vi "Rate scan x8.vi"(6 "T Ventana":u32 format="%x", 7 "Espera acceso USB":u32, 8 "error in 2":errorcluster, 9 "Valor buscado scalers (5000)":u16, 10 "Sumador":u8, 11 "ftHandle_in 2":u32) -> (0 "error out 2":errorcluster, 1 "DAC\nTH3,TH4,TH5":u16, 2 "DAC\nTH0,TH1,TH2":u16, 3 "ftHandle_out 2":u32, 5 "Scaler 1":u16)   [LabVIEW 2009]
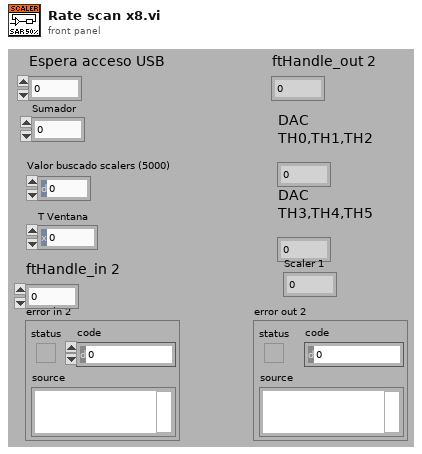
[diagram p1: front panel]
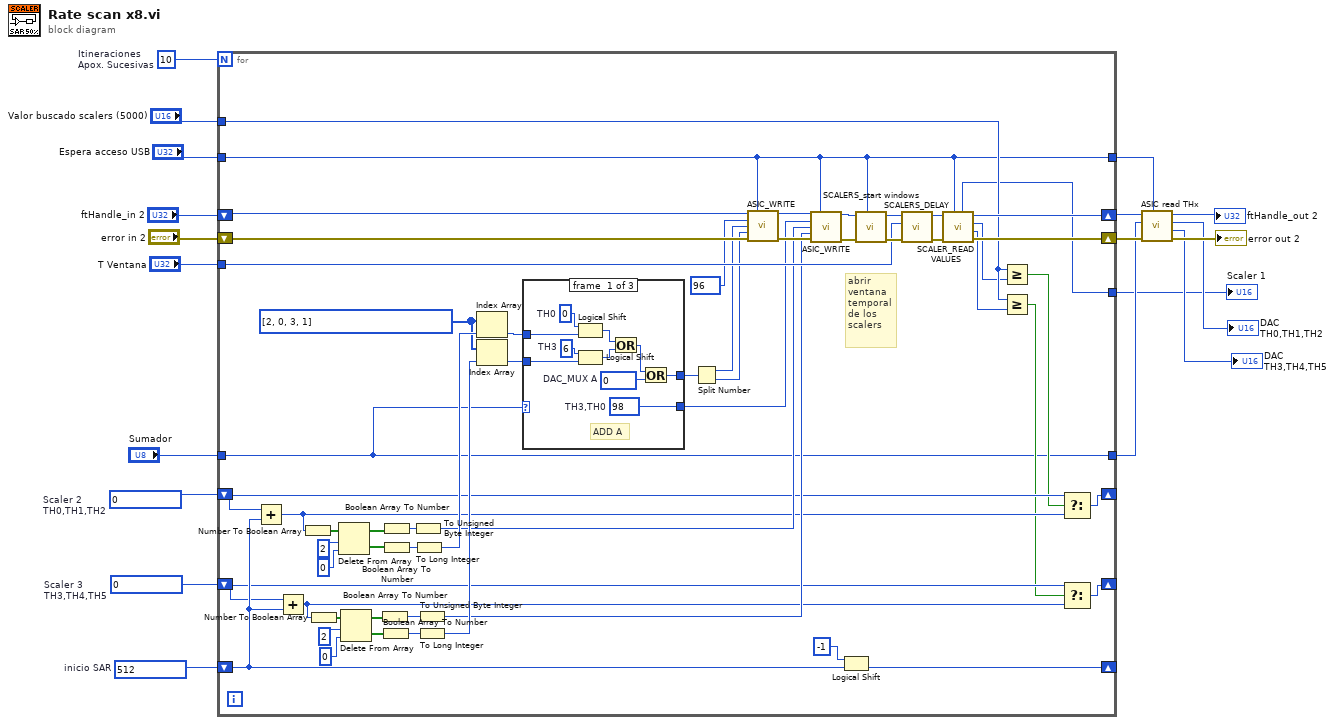
[diagram p0: block diagram]
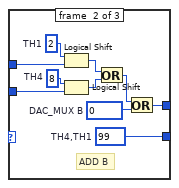
[diagram p2: hidden frame]
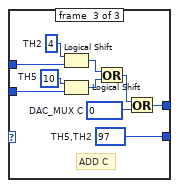
[diagram p3: hidden frame]
diagram:
  w11 = u16 0  # Scaler 3 TH3,TH4,TH5
  w12 = u16 0  # Scaler 2 TH0,TH1,TH2
  w13 = u16 512  # inicio SAR
  w15 = 10  # Itineraciones Apox. Sucesivas
  n1 = for {
    N: w15 -> [_]
    tunnel: "Espera acceso USB" -> [w21]
    tunnel: "T Ventana" -> [w73]
    tunnel: "Valor buscado scalers (5000)" -> [w23]
    shift-right: [w69] -> _
    shift-left: w13 -> [w68]
    shift-right: [w28] -> _
    shift-left: w12 -> [w35]
    shift-right: [w27] -> _
    shift-left: w11 -> [w33]
    tunnel: "Sumador" -> [w25]
    shift-right: [w30] -> w8
    shift-left: "ftHandle_in 2" -> [w51]
    shift-right: [w29] -> w9
    shift-left: "error in 2" -> [w50]
    tunnel: [w25] -> w6
    tunnel: [w21] -> w7
    tunnel: [w20] -> w1
    w48 = u16[] [2, 0, 3, 1]
    # "abrir ventana temporal de los scalers"
    n2 = Add(x=w35, y=w68) -> (x+y=w34:u16)
    n3 = Add(x=w33, y=w68) -> (x+y=w32:u16)
    n4 = Number To Boolean Array(number=w34) -> (Boolean array=w67:bool[])
    n5 = Number To Boolean Array(number=w32) -> (Boolean array=w66:bool[])
    n6 = Delete From Array(array=w67, length=2, index=0) -> (deleted portion=w60:bool[], array with subset deleted=w65:bool[])
    n7 = Delete From Array(array=w66, length=2, index=0) -> (deleted portion=w58:bool[], array with subset deleted=w59:bool[])
    n8 = Boolean Array To Number(Boolean array=w59) -> (number=w56:u32)
    n9 = Boolean Array To Number(Boolean array=w58) -> (number=w54:u32)
    n10 = Boolean Array To Number(Boolean array=w65) -> (number=w57:u32)
    n11 = Boolean Array To Number(Boolean array=w60) -> (number=w55:u32)
    n12 = To Unsigned Byte Integer(number=w57) -> (unsigned 8bit integer=w39:u8)
    n13 = To Long Integer(number=w55) -> (32bit integer=w53:i32)
    n14 = To Unsigned Byte Integer(number=w56) -> (unsigned 8bit integer=w38:u8)
    n15 = To Long Integer(number=w54) -> (32bit integer=w52:i32)
    n16 = Index Array(array=w48, index=w53) -> (element=w47:u16)
    n17 = Index Array(array=w48, index=w52) -> (element=w46:u16)
    n18 = case shown="0, Default" w25 {
      tunnel: [w85 w95 w105] -> w40
      tunnel: w47 -> [w84 w94 w104]
      tunnel: w46 -> [w83 w93 w103]
      tunnel: [w77 w87 w97] -> w41
      frame #0 {
        w76 = u16 0  # DAC_MUX A
        w81 = i8 6  # TH3
        w82 = i8 0  # TH0
        w85 = u8 98  # TH3,TH0
        # "ADD A"
        n19 = Logical Shift(y=w82, x=w84) -> (x << y=w79:u16)
        n20 = Logical Shift(y=w81, x=w83) -> (x << y=w80:u16)
        n21 = Or(x=w79, y=w80) -> (x .or. y?=w78:u16)
        n22 = Or(x=w78, y=w76) -> (x .or. y?=w77:u16)
      }
      frame #1 {
        w86 = u16 0  # DAC_MUX B
        w91 = i8 8  # TH4
        w92 = i8 2  # TH1
        w95 = u8 99  # TH4,TH1
        # "ADD B"
        n23 = Logical Shift(y=w92, x=w94) -> (x << y=w89:u16)
        n24 = Logical Shift(y=w91, x=w93) -> (x << y=w90:u16)
        n25 = Or(x=w89, y=w90) -> (x .or. y?=w88:u16)
        n26 = Or(x=w88, y=w86) -> (x .or. y?=w87:u16)
      }
      frame #2 {
        w96 = u16 0  # DAC_MUX C
        w101 = i8 10  # TH5
        w102 = i8 4  # TH2
        w105 = u8 97  # TH5,TH2
        # "ADD C"
        n27 = Logical Shift(y=w102, x=w104) -> (x << y=w99:u16)
        n28 = Logical Shift(y=w101, x=w103) -> (x << y=w100:u16)
        n29 = Or(x=w99, y=w100) -> (x .or. y?=w98:u16)
        n30 = Or(x=w98, y=w96) -> (x .or. y?=w97:u16)
      }
    }
    n31 = Split Number(x=w41) -> (hi(x)=w42:u8, lo(x)=w43:u8)
    n32 = call "ASIC_WRITE.vi"("ftHandle_in"=w51, "Espera acceso USB"=w21, "Direccion Registro Asic"=u8 96, "Byte Alto"=w42, "Byte Bajo"=w43, "error in"=w50) -> ("ftHandle_out"=w45:u32, "error out"=w44:errorcluster)  [unwired: 8 in]
    n33 = call "ASIC_WRITE.vi"("ftHandle_in"=w45, "Espera acceso USB"=w21, "Direccion Registro Asic"=w40, "Byte Alto"=w39, "Byte Bajo"=w38, "error in"=w44) -> ("ftHandle_out"=w37:u32, "error out"=w36:errorcluster)  [unwired: 8 in]
    n34 = Logical Shift(y=i8 -1, x=w68) -> (x << y=w69:u16)
    n35 = call "SCALERS_start windows.vi"("Espera acceso USB"=w21, "error in 2"=w36, "ftHandle_in 2"=w37) -> ("error out"=w74:errorcluster, "ftHandle_out"=w75:u32)  [unwired: 7 in]
    n36 = call "SCALERS_DELAY.vi"("error out 2"=w74, "Ventana 2"=w73, "ftHandle_out 2"=w75) -> ("error out"=w71:errorcluster, "ftHandle_out"=w72:u32)  [unwired: 7 in]
    n37 = call "SCALER_READ VALUES.vi"("Espera acceso USB"=w21, "error in"=w71, "ftHandle_in"=w72) -> ("error out"=w29:errorcluster, "Scaler 3"=w24:u16, "Scaler 2"=w22:u16, "ftHandle_out"=w30:u32, "Scaler 1"=w20:u16)  [unwired: 3 in, 1 out]
    n38 = Greater Or Equal?(x=w23, y=w22) -> (x >= y?=w31:bool)
    n39 = Greater Or Equal?(x=w23, y=w24) -> (x >= y?=w26:bool)
    n40 = Select(t=w35, s=w31, f=w34) -> (s? t:f=w28:u16)
    n41 = Select(t=w33, s=w26, f=w32) -> (s? t:f=w27:u16)
  }
  "Scaler 1" <- w1
  n42 = call "ASIC read THx.vi"("Espera acceso USB"=w7, "error in"=w9, "Sumador"=w6, "ftHandle_in"=w8) -> ("error out 2"=→"error out 2":errorcluster, "THx+3"=→"DAC\nTH3,TH4,TH5":u16, "THx"=→"DAC\nTH0,TH1,TH2":u16, "ftHandle_out 2"=→"ftHandle_out 2":u32)  [unwired: 4 in]
